vi "mux2.vi"(0 "MUX S.n.":string, 2 "Switch":u16(ring) items=["Wagner", "Ground"], 3 "error in (no error)":errorcluster) -> (8 "error out":errorcluster)   [LabVIEW 2014]
uses:
  <vilib>/Utility/config.llb/Read Key (String).vi
  <vilib>/Utility/config.llb/NI_LVConfig.lvlib
panel:
  out "ext.cmd":string=" -b"
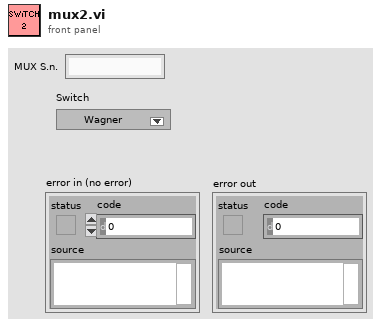
[diagram p1: front panel]
types:
  T1 = typedef "NI_LVConfig.lvlib/Config Data RefNum.ctl" = refnum<k1>
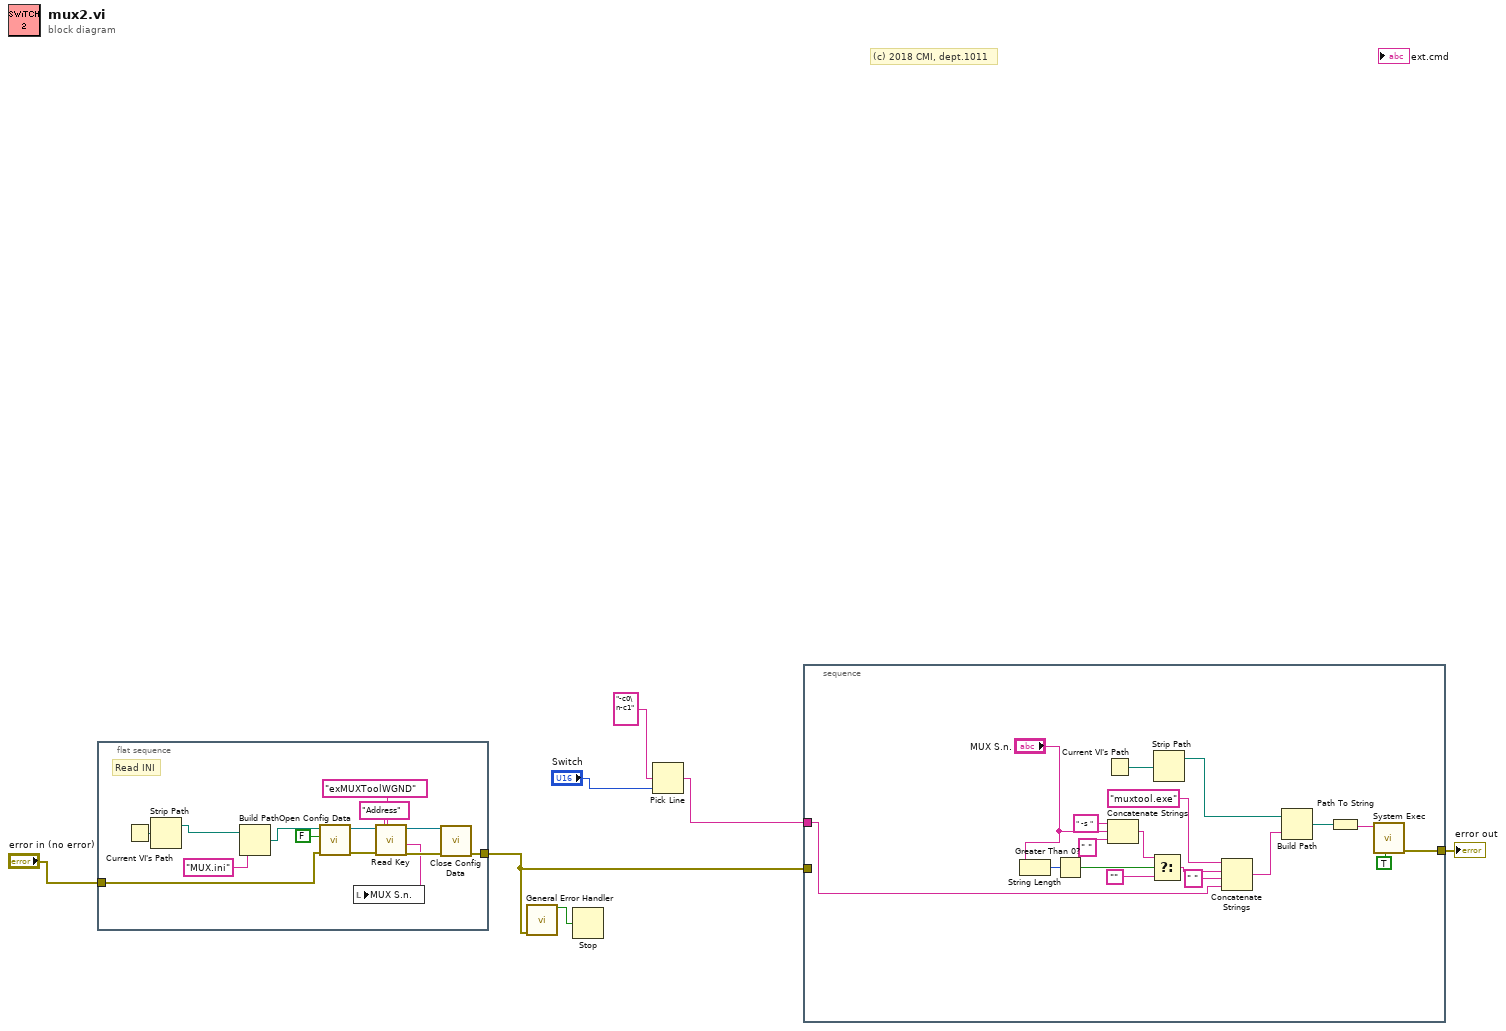
[diagram p0: block diagram]
diagram:
  # "(c) 2018 CMI, dept.1011"
  n1 = flat-sequence {
    tunnel: [w12] -> w4
    tunnel: "error in (no error)" -> [w8]
    frame #0 {
      # "Read INI"
      n2 = Current VI's Path() -> (path=w10:path)
      n3 = Strip Path(path=w10) -> (stripped path=w9:path)  [unwired: 1 out]
      n4 = Build Path(base path=w9, name or relative path="MUX.ini") -> (appended path=w20:path)
      n5 = call <vilib>:"Open Config Data.vi"("error in (no error)"=w8, "create file if necessary (T)"=FALSE, "configuration file path"=w20) -> ("error out"=w18:errorcluster, "refnum"=w11:T1)  [unwired: 6 in, 1 out]
      n6 = call-poly <vilib>:"Read Key.vi"("section"="exMUXToolWGND", "error in (no error)"=w18, "key"="Address", "refnum"=w11) -> ("error out"=w14:errorcluster, "value"=w13:string, "refnum out"=w15:T1)  [unwired: 4 in, 1 out]
      n7 = local write "MUX S.n."(w13) -> ()
      n8 = call <vilib>:"Close Config Data.vi"("error in (no error)"=w14, "refnum"=w15) -> ("error out"=w12:errorcluster)  [unwired: 8 in, 1 out]
    }
  }
  n9 = call <vilib>:"General Error Handler.vi"("error in (no error)"=w4) -> ("error?"=w7:bool)  [unwired: 10 in, 4 out]
  n10 = Stop(stop? (T)=w7) -> ()
  n11 = Pick Line(multi-line string="-c0\n-c1", line index="Switch") -> (output string=w5:string)  [unwired: 1 in]
  n12 = stacked-sequence {
    tunnel: w5 -> [w23]
    tunnel: w4 -> [_]
    tunnel: [w22] -> w2
    frame #0 {
      n13 = String Length(string="MUX S.n.") -> (length=w30:i32)
      n14 = Greater Than 0?(x=w30) -> (x > 0?=w29:bool)
      n15 = Current VI's Path() -> (path=w37:path)
      n16 = Concatenate Strings(" -s " ("string"), "MUX S.n.", " " ("string")) -> (w26:string)
      n17 = Select(t=w26, s=w29, f="") -> (s? t:f=w31:string)
      n18 = Strip Path(path=w37) -> (stripped path=w36:path)  [unwired: 1 out]
      n19 = Concatenate Strings("muxtool.exe" ("name or relative path"), w31, " " ("string"), w23) -> (w33:string)
      n20 = Build Path(base path=w36, name or relative path=w33) -> (appended path=w39:path)
      n21 = Path To String(path=w39) -> (string=w38:string)
      n22 = call <vilib>:"System Exec.vi"("run minimized? (F)"=TRUE, "command line"=w38) -> ("error out"=w22:errorcluster)  [unwired: 6 in, 3 out]
    }
  }
  "error out" <- w2
